vi "CRYReplace Default Names.vi"(11 "Analysis In":T1={"Name"="", "Harmonics"=[1.0], " Algorithm"=0, "delay"=0.0, "THD(%)"=FALSE, "Rub&Buzz"=FALSE, "Imp"=FALSE, "Imp Ref resistor"=1.0, "Y data"=0, "Y prefix"="", "Y unit"="", "Y dB ref"=1.0, "Custom Curve Names"=[], "har list items"=[""], "Envelope"=FALSE, "use custom unit"=FALSE, "autodelay ch"=0.0, "impulse"=FALSE, " start ms"=1.0, " stop ms"=1.0, "Scaling"=1, "Default Overlap "=FALSE, "Advanced View"=FALSE, "Loose Particle"=FALSE, "Use default"=FALSE, "Auto-Correlation(Stimulus)"=FALSE, "Auto-Correlation(Response)"=FALSE, "Deconvolved Response"=FALSE, "Mic Current"=FALSE, "M List Vaiues"=0, "Type"=0, "Delay Method"=3, "Apply Correction Out"=FALSE, "Apply Correction In"=FALSE, "Harmonics @ meas.frq"=FALSE, "THD Normalized(%)"=FALSE, "Total Distortion"=FALSE, "THD+Noise(%)"=FALSE, "Rub&Buzz Norm'd(%)"=FALSE, "Standard Error"=FALSE, "Confidence Limits"=FALSE, "Total Diff"=FALSE, "Total Noise"=FALSE, "Total DFD(%)"=FALSE, "Total IMD(%)"=FALSE, "Total IM"=FALSE, "Total DFD+Noise(%)"=FALSE, "Use Channel Name"=FALSE, "Waveform In"="", "Waveform Out"="", "Method"=3, "Spectral Scaling"=3, "Appliied Unit"=1, "Length Unit"=1, "Applied Units"=1, "Sens Item"=0, "Tab"=1, "Distance Unit"=0, "discard cycles"=1.0, "Weigting"="", "Averaging Time"=0.0, "Max duration"=0.0, "Min duration"=0.0, "Attack Threshold"=0.0, "Hysteresis Up"=0.0, "Fmin(Hz)"=0.0, "Fmax(Hz)"=0.0, "Freq.Resolution"=0.0, "Over-samples Res."=0.0, "Win Resolution"=0.0, "distance"=0.0, "samples"=1.0, "Overlap"=1.0, "Record Length"=1.0, "No.of FFTs"=0.0, "Hz"=1.0, "record delay"=1.0, " Std Err"=1.0, "Response"=FALSE, "Coherent Power*"=FALSE, "Stimulus"=FALSE, "Measurement Confidence"=FALSE, "Auto Spectrum(Response)*"=FALSE, "Auto Spectrum(Stimulus)*"=FALSE, "Cross Spectrum*"=FALSE, "functions"=FALSE, "Frequency Response"=FALSE, "Non-Coherent Power*"=FALSE, "Coherence (%)"=FALSE, "Non-Coherence (%)"=FALSE, "Signal-Noise Ratio (dB)"=FALSE, "Non-Coherenct Distirtion*"=FALSE, "Result Waveforms"=FALSE, "Coupling"=FALSE, "Averaging"=0, "Harmonics"=0, "Custom Curve Names"=0, "unLabel"="", "Custom Curve Names"="", "Unit"="", "Total IMD + Noise(%) "=FALSE, "ResponseMe"=1, "Intermod"=[1.0], "Diff\n"=[1.0], "Cross-Correlation"=FALSE, "IM list items"=[""], "Diff list items"=[""], "TSR Window Type"="", "Help"="", "Custom Curve IDs"=[], "Default Curve Names"=[], "Loose Particle waveform"=FALSE, "Perceptual Rub&Buzz"=FALSE, "Imp Auto Mode"=0, "Mic Auto Mode"=0, "Mic Ref resistor"=1.0, "Curve Resolution"=3, "Curve Resolution Hz"=0.0, "Polarity"=FALSE} {"Curve Resolution Hz" format="%.2f"; "Mic Ref resistor" format="%.2f"; "Diff" format="%.2f"; "Intermod" format="%.2f"; "ResponseMe" items=["Absolute", "Relative"]; "Std Err" format="%.1f"; "record delay" format="%.1f"; "Hz" format="%.1f"; "No.of FFTs" format="%.2f"; "Record Length" format="%.1f"; "Overlap" format="%.1f"; "samples" format="%.1f"; "distance" format="%.2f"; "Win Resolution" format="%.2f"; "Over-samples Res." format="%.2f"; "Freq.Resolution" format="%.2f"; "Fmax(Hz)" format="%.2f"; "Fmin(Hz)" format="%.2f"; "Hysteresis Up" format="%.2f"; "Attack Threshold" format="%.2f"; "Min duration" format="%.2f"; "Max duration" format="%.2f"; "Averaging Time" format="%.2f"; "Distance Unit" items=["Absolute", "Relative"]; "Sens Item" items=["x", "y", "z"]; "Applied Units" items=["Absolute", "Relative"]; "Length Unit" items=["Absolute", "Relative"]; "Appliied Unit" items=["Absolute", "Relative"]; "Spectral Scaling" items=["Absolute", "Relative"]; "M List Vaiues" items=["x", "y", "z"]; "Scaling" format="%.1f"; "stop ms" format="%.1f"; "start ms" format="%.1f"; "Y data" items=["dB", "Lin"]; "Y dB ref" format="%.1f"; "Imp Ref resistor" format="%.2f"; "Harmonics" format="%.2f"; "delay" format="%.2f"}) -> (3 "Analysis Out":T1={"Name"="", "Harmonics"=[1.0], " Algorithm"=0, "delay"=0.0, "THD(%)"=FALSE, "Rub&Buzz"=FALSE, "Imp"=FALSE, "Imp Ref resistor"=1.0, "Y data"=0, "Y prefix"="", "Y unit"="", "Y dB ref"=1.0, "Custom Curve Names"=[], "har list items"=[""], "Envelope"=FALSE, "use custom unit"=FALSE, "autodelay ch"=0.0, "impulse"=FALSE, " start ms"=1.0, " stop ms"=1.0, "Scaling"=1, "Default Overlap "=FALSE, "Advanced View"=FALSE, "Loose Particle"=FALSE, "Use default"=FALSE, "Auto-Correlation(Stimulus)"=FALSE, "Auto-Correlation(Response)"=FALSE, "Deconvolved Response"=FALSE, "Mic Current"=FALSE, "M List Vaiues"=0, "Type"=0, "Delay Method"=3, "Apply Correction Out"=FALSE, "Apply Correction In"=FALSE, "Harmonics @ meas.frq"=FALSE, "THD Normalized(%)"=FALSE, "Total Distortion"=FALSE, "THD+Noise(%)"=FALSE, "Rub&Buzz Norm'd(%)"=FALSE, "Standard Error"=FALSE, "Confidence Limits"=FALSE, "Total Diff"=FALSE, "Total Noise"=FALSE, "Total DFD(%)"=FALSE, "Total IMD(%)"=FALSE, "Total IM"=FALSE, "Total DFD+Noise(%)"=FALSE, "Use Channel Name"=FALSE, "Waveform In"="", "Waveform Out"="", "Method"=3, "Spectral Scaling"=3, "Appliied Unit"=1, "Length Unit"=1, "Applied Units"=1, "Sens Item"=0, "Tab"=1, "Distance Unit"=0, "discard cycles"=1.0, "Weigting"="", "Averaging Time"=0.0, "Max duration"=0.0, "Min duration"=0.0, "Attack Threshold"=0.0, "Hysteresis Up"=0.0, "Fmin(Hz)"=0.0, "Fmax(Hz)"=0.0, "Freq.Resolution"=0.0, "Over-samples Res."=0.0, "Win Resolution"=0.0, "distance"=0.0, "samples"=1.0, "Overlap"=1.0, "Record Length"=1.0, "No.of FFTs"=0.0, "Hz"=1.0, "record delay"=1.0, " Std Err"=1.0, "Response"=FALSE, "Coherent Power*"=FALSE, "Stimulus"=FALSE, "Measurement Confidence"=FALSE, "Auto Spectrum(Response)*"=FALSE, "Auto Spectrum(Stimulus)*"=FALSE, "Cross Spectrum*"=FALSE, "functions"=FALSE, "Frequency Response"=FALSE, "Non-Coherent Power*"=FALSE, "Coherence (%)"=FALSE, "Non-Coherence (%)"=FALSE, "Signal-Noise Ratio (dB)"=FALSE, "Non-Coherenct Distirtion*"=FALSE, "Result Waveforms"=FALSE, "Coupling"=FALSE, "Averaging"=0, "Harmonics"=0, "Custom Curve Names"=0, "unLabel"="", "Custom Curve Names"="", "Unit"="", "Total IMD + Noise(%) "=FALSE, "ResponseMe"=1, "Intermod"=[1.0], "Diff\n"=[1.0], "Cross-Correlation"=FALSE, "IM list items"=[""], "Diff list items"=[""], "TSR Window Type"="", "Help"="", "Custom Curve IDs"=[], "Default Curve Names"=[], "Loose Particle waveform"=FALSE, "Perceptual Rub&Buzz"=FALSE, "Imp Auto Mode"=0, "Mic Auto Mode"=0, "Mic Ref resistor"=1.0, "Curve Resolution"=3, "Curve Resolution Hz"=0.0, "Polarity"=FALSE} {"Curve Resolution Hz" format="%.2f"; "Mic Ref resistor" format="%.2f"; "Diff" format="%.2f"; "Intermod" format="%.2f"; "ResponseMe" items=["Absolute", "Relative"]; "Std Err" format="%.1f"; "record delay" format="%.1f"; "Hz" format="%.1f"; "No.of FFTs" format="%.2f"; "Record Length" format="%.1f"; "Overlap" format="%.1f"; "samples" format="%.1f"; "distance" format="%.2f"; "Win Resolution" format="%.2f"; "Over-samples Res." format="%.2f"; "Freq.Resolution" format="%.2f"; "Fmax(Hz)" format="%.2f"; "Fmin(Hz)" format="%.2f"; "Hysteresis Up" format="%.2f"; "Attack Threshold" format="%.2f"; "Min duration" format="%.2f"; "Max duration" format="%.2f"; "Averaging Time" format="%.2f"; "Distance Unit" items=["Absolute", "Relative"]; "Sens Item" items=["x", "y", "z"]; "Applied Units" items=["Absolute", "Relative"]; "Length Unit" items=["Absolute", "Relative"]; "Appliied Unit" items=["Absolute", "Relative"]; "Spectral Scaling" items=["Absolute", "Relative"]; "M List Vaiues" items=["x", "y", "z"]; "Scaling" format="%.1f"; "stop ms" format="%.1f"; "start ms" format="%.1f"; "Y data" items=["dB", "Lin"]; "Y dB ref" format="%.1f"; "Imp Ref resistor" format="%.2f"; "Harmonics" format="%.2f"; "delay" format="%.2f"})   [LabVIEW 2013]
uses:
  Typedef Control/CRYAnalysis Cluster.ctl
  Calibration/SubVI/CRYCal Global.vi
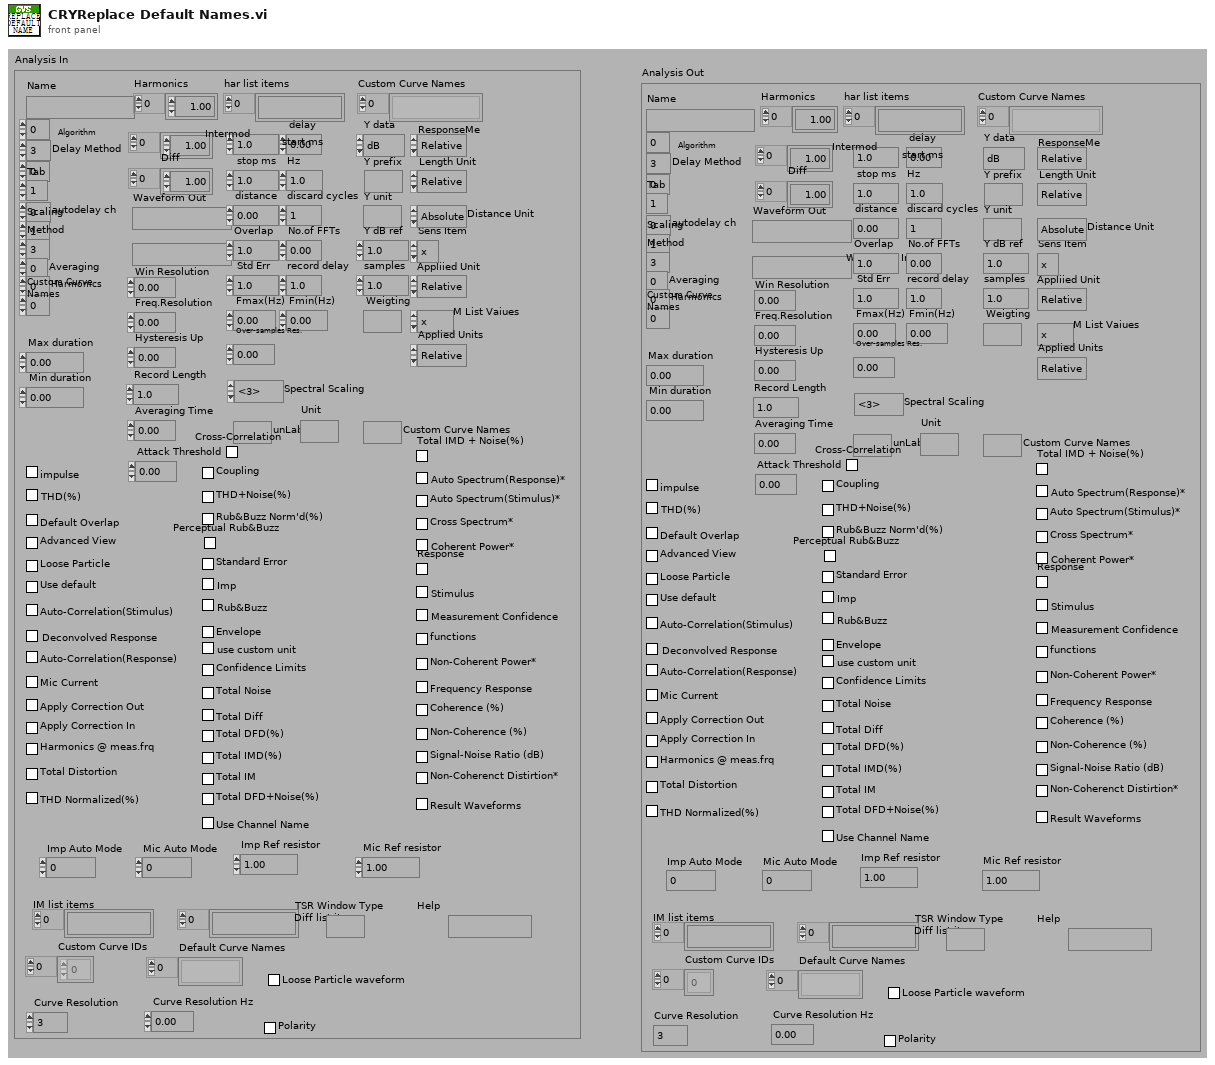
[diagram p1: front panel]
types:
  T1 = typedef "CRYAnalysis Cluster.ctl" = cluster{"Name":string, "Harmonics":dbl[], " Algorithm":u16, "delay":dbl, "THD(%)":bool, "Rub&Buzz":bool, "Imp":bool, "Imp Ref resistor":dbl, "Y data":u16, "Y prefix":string, "Y unit":string, "Y dB ref":dbl, "Custom Curve Names":string[], "har list items":string[], "Envelope":bool, "use custom unit":bool, "autodelay ch":dbl, "impulse":bool, " start ms":dbl, " stop ms":dbl, "Scaling":i32, "Default Overlap ":bool, "Advanced View":bool, "Loose Particle":bool, "Use default":bool, "Auto-Correlation(Stimulus)":bool, "Auto-Correlation(Response)":bool, "Deconvolved Response":bool, "Mic Current":bool, "M List Vaiues":u16, "Type":u16, "Delay Method":u16, "Apply Correction Out":bool, "Apply Correction In":bool, "Harmonics @ meas.frq":bool, "THD Normalized(%)":bool, "Total Distortion":bool, "THD+Noise(%)":bool, "Rub&Buzz Norm'd(%)":bool, "Standard Error":bool, "Confidence Limits":bool, "Total Diff":bool, "Total Noise":bool, "Total DFD(%)":bool, "Total IMD(%)":bool, "Total IM":bool, "Total DFD+Noise(%)":bool, "Use Channel Name":bool, "Waveform In":string, "Waveform Out":string, "Method":u16, "Spectral Scaling":u16, "Appliied Unit":u16, "Length Unit":u16, "Applied Units":u16, "Sens Item":u16, "Tab":i32, "Distance Unit":u16, "discard cycles":dbl, "Weigting":string, "Averaging Time":dbl, "Max duration":dbl, "Min duration":dbl, "Attack Threshold":dbl, "Hysteresis Up":dbl, "Fmin(Hz)":dbl, "Fmax(Hz)":dbl, "Freq.Resolution":dbl, "Over-samples Res.":dbl, "Win Resolution":dbl, "distance":dbl, "samples":dbl, "Overlap":dbl, "Record Length":dbl, "No.of FFTs":dbl, "Hz":dbl, "record delay":dbl, " Std Err":dbl, "Response":bool, "Coherent Power*":bool, "Stimulus":bool, "Measurement Confidence":bool, "Auto Spectrum(Response)*":bool, "Auto Spectrum(Stimulus)*":bool, "Cross Spectrum*":bool, "functions":bool, "Frequency Response":bool, "Non-Coherent Power*":bool, "Coherence (%)":bool, "Non-Coherence (%)":bool, "Signal-Noise Ratio (dB)":bool, "Non-Coherenct Distirtion*":bool, "Result Waveforms":bool, "Coupling":bool, "Averaging":u16, "Harmonics":i32, "Custom Curve Names":i32, "unLabel":string, "Custom Curve Names":string, "Unit":string, "Total IMD + Noise(%) ":bool, "ResponseMe":u16, "Intermod":dbl[], "Diff\n":dbl[], "Cross-Correlation":bool, "IM list items":string[], "Diff list items":string[], "TSR Window Type":string, "Help":string, "Custom Curve IDs":i32[], "Default Curve Names":string[], "Loose Particle waveform":bool, "Perceptual Rub&Buzz":bool, "Imp Auto Mode":u16, "Mic Auto Mode":u16, "Mic Ref resistor":dbl, "Curve Resolution":u16, "Curve Resolution Hz":dbl, "Polarity":bool}
  T2 = cluster{"Custom Curve Names":string, "Custom Curve IDs":i32, "Default Curve Names":string}[]
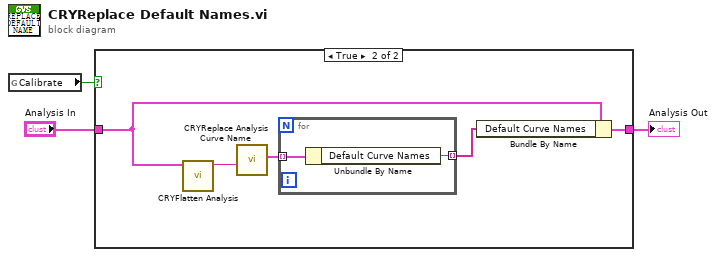
[diagram p0: block diagram]
diagram:
  n1 = global read "CRYCal Global.vi" "Calibrate"() -> (w3:bool)
  n2 = case shown="True" w3 {
    tunnel: "Analysis In" -> [w4 w8]
    tunnel: [w4 w5] -> w1
    frame False {
    }
    frame True {
      n3 = call "CRYFlatten Analysis.vi"("Analysis"=w8) -> ("Analysis flattened"=w7:string)  [unwired: 10 in]
      n4 = call "CRYReplace Analysis Curve Name.vi"("Step Setup In"=w7) -> ("Curve Info Array Out"=w6:T2)  [unwired: 6 in, 4 out]
      n5 = for {
        tunnel: w6 -> [w11] mode=indexing
        tunnel: [w10] -> w9 mode=indexing
        n6 = Unbundle By Name(w11) -> ("Default Curve Names"=w10:string)
      }
      n7 = Bundle By Name(cluster=w8, "Default Curve Names"=w9) -> (w5:T1)
    }
  }
  "Analysis Out" <- w1
